vi "IO_DataQ_BuildInitMsg.vi"(9 "Filter":bool=TRUE, 10 "Num Chan":i32=2, 11 "Command List":string="srate 6000\nps 2\ndec 100\ndeca 1\nnop\n") -> (3 "Array":string[](array[string]))   [LabVIEW 2024]
panel:
  # "PS = 2     64 byte packet size\nSample Rate = 60,000,000/(srate * dec * deca)"
  # "srate 6000\nps 2\ndec 100\ndeca 1\nnop"
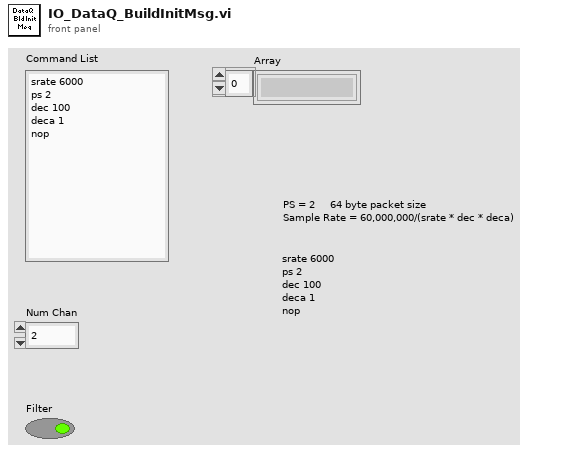
[diagram p1: front panel]
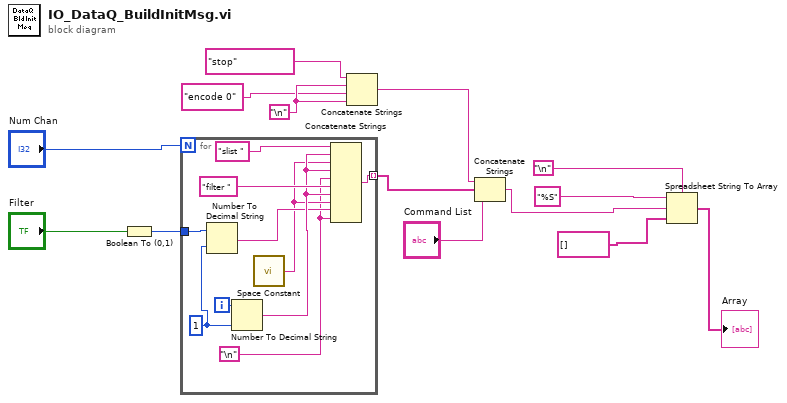
[diagram p0: block diagram]
diagram:
  w14 = "\n"
  n1 = Boolean To (0,1)(Boolean="Filter") -> (0, 1=w10:i16)
  n2 = for {
    N: "Num Chan" -> [_]
    tunnel: [w23] -> w6 mode=indexing
    tunnel: w10 -> [w21]
    i -> [w22]
    w15 = "\n"
    w18 = i16 1 ("width (-)")
    n3 = Number To Decimal String(number=w21, width (-)=w18) -> (decimal integer string=w17:string)
    n4 = Number To Decimal String(number=w22, width (-)=w18) -> (decimal integer string=w19:string)
    n5 = call <vilib>:"Space Constant.vi"() -> ("String"=w16:string)
    n6 = Concatenate Strings("slist ", w19, w16, w19, w15, "filter ", w19, w16, w17, w15) -> (w23:string)
  }
  n7 = Concatenate Strings("stop" ("Command List 2"), w14, "encode 0" ("Command List 2"), w14) -> (w11:string)
  n8 = Concatenate Strings(w11, w6, "Command List") -> (w7:string)
  n9 = Spreadsheet String To Array(delimiter (Tab)="\n", format string="%S", spreadsheet string=w7, array type (2D Dbl)=string[] []) -> (array=→"Array":string[])
